vi "Write Data.vi"(10 "数据":i32, 11 "Task A任务消息输入":refnum<class "Task A任务消息.lvclass">) -> (3 "Task A任务消息输出":refnum<class "Task A任务消息.lvclass">)   [LabVIEW 2013, in "Task A操作者.lvlib" / "Task A任务消息.lvclass"]
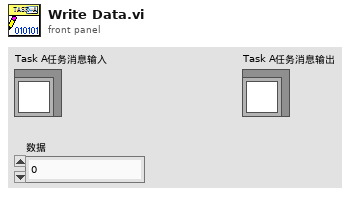
[diagram p1: front panel]
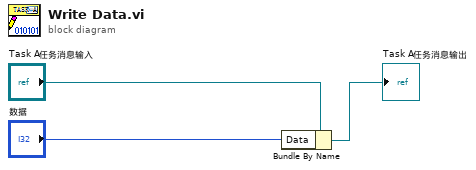
[diagram p0: block diagram]
diagram:
  n1 = Bundle By Name(cluster="Task A任务消息输入", "Data"="数据") -> (→"Task A任务消息输出":refnum<class "Task A任务消息.lvclass">)
